vi "SSC Digital PPMU Configure Current Limit Range.vi"(0 "Digital SSC in":T1[](array[typedef]), 5 "Current Limit Range (A)":dbl format="%#_6p", 11 "error in":errorcluster) -> (4 "Digital SSC out":T1[](array[typedef]), 15 "error out":errorcluster)   [LabVIEW 2019]
doc: "Specifies the current limit range for the specified pin(s) and pin group(s) when forcing voltage. You must call the PPMU Source VI for changes to the PPMU configuration to take effect, even if the PPMU is already sourcing."
uses:
  SSC Digital.ctl
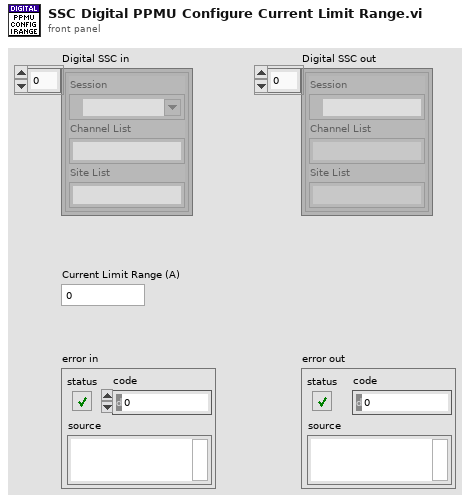
[diagram p1: front panel]
types:
  T1 = typedef "SSC Digital.ctl" = cluster{"Session":refnum<k15>, "Channel List":string, "Site List":string}
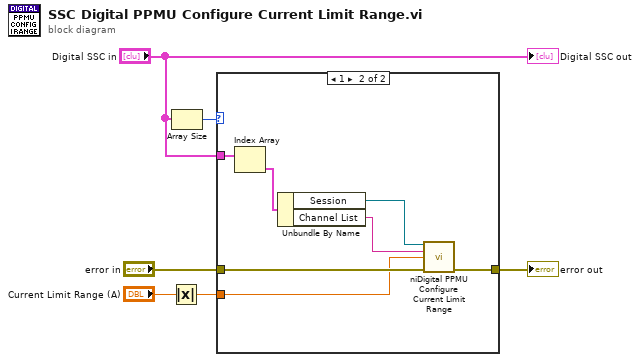
[diagram p0: block diagram]
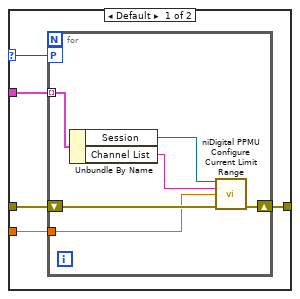
[diagram p2: hidden frame]
diagram:
  n1 = Absolute Value(x="Current Limit Range (A)") -> (abs(x)=w4:dbl)
  n2 = Array Size(array="Digital SSC in") -> (size(s)=w2:i32)
  n3 = case shown="1" w2 {
    selector: w2 -> [w8 _]
    tunnel: "error in" -> [w11 w24]
    tunnel: w4 -> [w10 w23]
    tunnel: [w9 w22] -> w3
    tunnel: "Digital SSC in" -> [w7 w21]
    frame Default {
      n4 = for {
        tunnel: w10 -> [w16]
        workers-P: w8 -> [_]
        tunnel: w7 -> [w15] mode=indexing
        shift-right: [w12] -> w9
        shift-left: w11 -> [w17]
        n5 = Unbundle By Name(w15) -> ("Session"=w14:refnum<k15>, "Channel List"=w13:string)
        n6 = call <instrlib>:"niDigital PPMU Configure Current Limit Range.vi"("instrument handle"=w14, "channel list"=w13, "current limit range (A)"=w16, "error in"=w17) -> ("error out"=w12:errorcluster)  [unwired: 10 in, 1 out]
      }
    }
    frame 1 {
      n7 = Index Array(array=w21) -> (element=w18:T1)  [unwired: 1 in]
      n8 = Unbundle By Name(w18) -> ("Session"=w20:refnum<k15>, "Channel List"=w19:string)
      n9 = call <instrlib>:"niDigital PPMU Configure Current Limit Range.vi"("instrument handle"=w20, "channel list"=w19, "current limit range (A)"=w23, "error in"=w24) -> ("error out"=w22:errorcluster)  [unwired: 10 in, 1 out]
    }
  }
  "error out" <- w3
  "Digital SSC out" <- "Digital SSC in"
